vi "getRotAng.vi"(8 "error in (no error)":errorcluster, 11 "CamRot in":refnum<class "CamRot.lvclass">) -> (0 "error out":errorcluster, 2 "Rotation Angle in Deg":dbl, 3 "CamRot out":refnum<class "CamRot.lvclass">)   [LabVIEW 2016, in "OfcFunc.lvlib" / "CamRot.lvclass"]
doc: "Get the rotation angle in degree."
uses:
  CamRot.lvclass
  CamRot.lvclass/CamRot.ctl
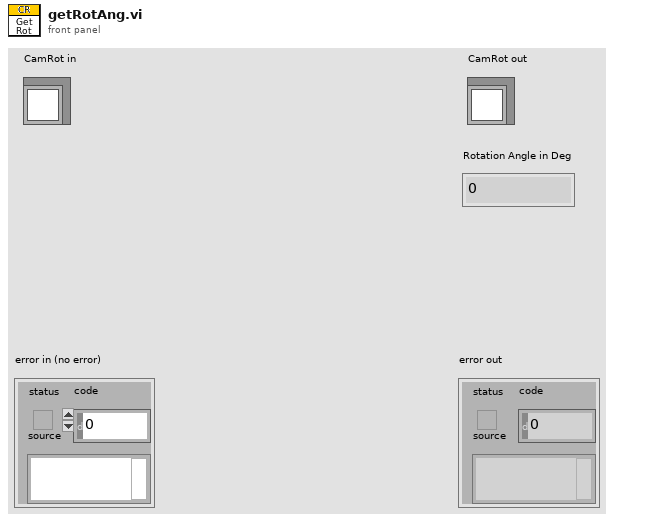
[diagram p1: front panel]
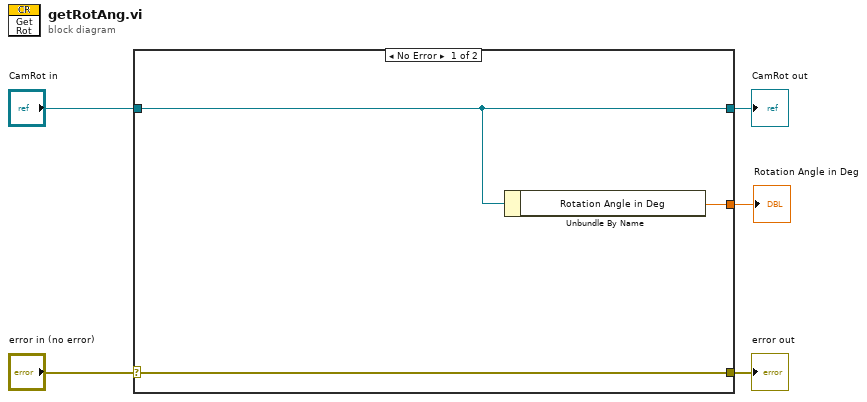
[diagram p0: block diagram]
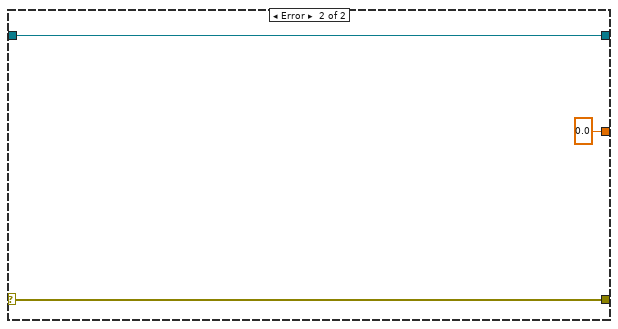
[diagram p2: hidden frame]
diagram:
  n1 = case shown="No Error" "error in (no error)" {
    selector: "error in (no error)" -> [w8 w11]
    tunnel: [w8 w11] -> w4
    tunnel: [w7 w10] -> w2
    tunnel: "CamRot in" -> [w7 w10]
    tunnel: [w6 0.0 ("Rotation Angle in Deg")] -> w1
    frame No Error {
      n2 = Unbundle By Name(w7) -> ("Rotation Angle in Deg"=w6:dbl)
    }
    frame Error {
    }
  }
  "error out" <- w4
  "CamRot out" <- w2
  "Rotation Angle in Deg" <- w1
